vi "readingfromfile.vi"() -> ()   [LabVIEW 2020]
uses:
  <vilib>/Instr/_visa.llb/VISA Configure Serial Port (Instr).vi
panel:
  out "error out":errorcluster
  out "return count":u32
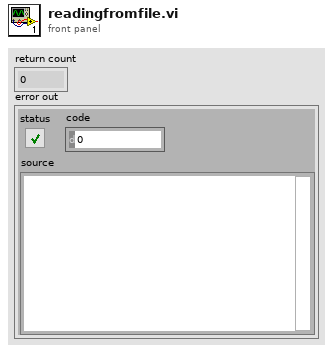
[diagram p1: front panel]
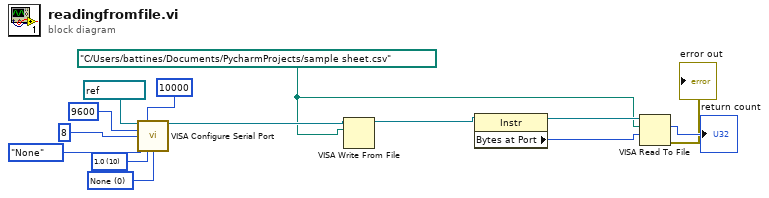
[diagram p0: block diagram]
diagram:
  w4 = path "C:/Users/battines/Documents/PycharmProjects/sample sheet.csv" ("filename")
  w9 = u16 0 items=["None", "XON/XOFF", "RTS/CTS", "XON/XOFF & RTS/CTS", "DTR/DSR", "XON/XOFF & DTR/DSR"] ("flow control (0:none)")
  w10 = u16 10 items=["1.0"=10, "1.5"=15, "2.0"=20] ("stop bits (10: 1 bit)")
  n1 = call-poly "VISA Configure Serial Port"("VISA resource name"=refnum<visa-resource-name> "COM3", "timeout (10sec)"=u32 10000, "baud rate (9600)"=u32 9600, "data bits (8)"=u16 8, "parity (0:none)"=enum16{"None", "Odd", "Even", "Mark", "Space"}."None", "stop bits (10: 1 bit)"=w10, "flow control (0:none)"=w9) -> ("VISA resource name out"=w7:refnum<visa-resource-name>)  [unwired: 7 in, 1 out]
  n2 = VISA Write From File(10:w4, 11:w7) -> (3:w6:refnum<visa-resource-name>)  [unwired: 2 in, 2 out]
  n3 = property class="Instr"(reference=w6) -> (reference out=w5:refnum<visa-resource-name>, "Bytes at Port"=w3:u32)  [unwired: 1 in, 1 out]
  n4 = VISA Read To File(9:w3, 10:w4, 11:w5) -> (0:→"error out":errorcluster, 2:→"return count":u32)  [unwired: 1 in, 1 out]
